vi "GUILib.simple boolean update nominal.vi"(0 "ctlRef":refnum<vi>, 2 "nominalValue":bool, 4 "valueStatus":T1, 5 "error in (no error)":errorcluster) -> (14 "ctlRef out":refnum<vi>, 19 "error out":errorcluster)   [LabVIEW 2012, in "GUILib.lvlib"]
doc: "updates the nominal value for a specific type of control"
uses:
  GUILib.lvlib
  UtilityLib/UtilityLib.valueStatus.ctl
  UtilityLib/UtilityLib.lvlib
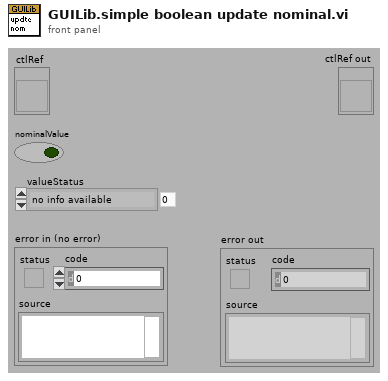
[diagram p1: front panel]
types:
  T1 = typedef "UtilityLib.lvlib/UtilityLib.valueStatus.ctl" = enum16{"no info available", "stand by/off", "on", "warning", "alarm/malfunction", "not implemented", "user action required", "important information", "system default", "control default", "indicator default", "button default"}
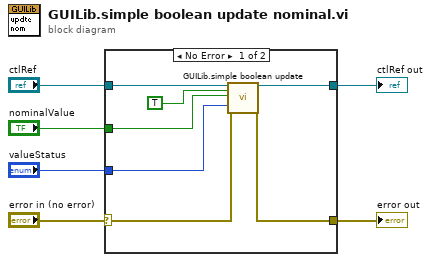
[diagram p0: block diagram]
diagram:
  n1 = case shown="No Error" "error in (no error)" {
    selector: "error in (no error)" -> [w9 w14]
    tunnel: [w8 w14] -> w5
    tunnel: "ctlRef" -> [w13 w15]
    tunnel: "valueStatus" -> [w11 _]
    tunnel: "nominalValue" -> [w10 _]
    tunnel: [w7 w15] -> w2
    frame No Error {
      n2 = call "GUILib.simple boolean update.vi"("ctlRef"=w13, "isNominal"=TRUE ("nominal"), "value"=w10, "valueStatus"=w11, "error in (no error)"=w9) -> ("ctlRef dup"=w7:refnum<vi>, "error out"=w8:errorcluster)  [unwired: 13 in]
    }
    frame Error {
    }
  }
  "ctlRef out" <- w2
  "error out" <- w5
